vi "Calibration.vi"(8 "error in (no error)":errorcluster) -> (0 "error out":errorcluster, 3 "V 2Pi\nActual":sgl=3.4309938 format="%#.1g")   [LabVIEW 2020]
uses:
  Controls/Calib states --- typedef.ctl
  <vilib>/vision/driver/NI_Vision_Acquisition_Software.lvlib
  <vilib>/vision/NI_Vision_Development_Module.lvlib
  Controls/Calib data ---typedef.ctl
  <vilib>/vision/Image Controls.llb/IMAQ Image.ctl
  64c00cdc-7401-4ced-a99b-d285ba44592a.vi
  Controls/Calibration color ---typedef.ctl
  Controls/LED panel ---typedef.ctl
  <vilib>/userDefined/High Color/IMAQdx.ctl
  Controls/Communication ports ---typedef.ctl
panel:
  out "Voltage range":i32 caption="Max voltage" format="%.0f V"
  out "Current Voltage":dbl format="%0.2f V"
  in  "Piezo voltage":dbl(slide) caption="Initial piezo voltage" min=0.0 max=75.0 step=0.01 scale=0.0..75.0 scale format="%#_2g"
  in  "V range":sgl=0.4 min=0.1 max=75 step=0.1 format="%.1f"
  in  "dt (ms)":i32=50 min=1 max=500 step=1
  in  "LED Panel":T1
  in  "Com ports":T2={"Piezo driver"="MDT694B", "Cam Session"="cam0", "Arduino"="COM7"}
  in  "Sust":bool=TRUE caption="Sustraer?"
  in  "dV (V)":sgl=0.4 min=0.1 max=5 step=0.1 format="%.1f"
  in  "Cancelar":bool
  in  "V 2Pi\nApriori":sgl=4.0 min=0.1 max=15 step=0.1 format="%.1f"
  out "valor enviado":string="17.2"
  in  "Iniciar":bool
  out "Captura":T4(plugin-control)
  out "tiempo total":u32=1016
  out "Ciclos 2Pi":cluster{"xi used":dbl[], "yi":dbl[]}[](graph)=[{"xi used"=[0.0, 0.4000000059604645, 0.800000011920929, 1.2000000476837158, 1.600000023841858, 2.0, 2.4000000953674316, 2.799999952316284, 3.200000047683716, 3.6000001430511475, 4.0, 4.400000095367432, 4.800000190734863, 5.200000286102295, 5.599999904632568, 6.0, 6.400000095367432, 6.800000190734863, 7.200000286102295], "yi"=[1.6194082498550415, 2.081223726272583, 3.9639101028442383, 5.417988300323486, 5.994996547698975, 5.763517379760742, 4.927460193634033, 3.268064022064209, 1.9228070974349976, 2.006049633026123, 3.322584629058838, 5.178757190704346, 5.874281883239746, 5.9817633628845215, 5.3586106300354, 3.7743194103240967, 2.4187028408050537, 2.3153183460235596, 3.7917206287384033]}, {"xi used"=[0.0, 0.10000000149011612, 0.20000000298023224, 0.30000000447034836, 0.4000000059604645, 0.5000000074505806, 0.6000000089406967, 0.7000000104308128, 0.800000011920929, 0.9000000208616257, 1.0000000298023224, 1.100000038743019, 1.2000000476837158, 1.3000000417232513, 1.4000000357627869, 1.5000000298023224, 1.600000023841858, 1.7000000178813934, 1.800000011920929, 1.9000000059604645, 2.0, 2.100000023841858, 2.200000047683716, 2.3000000715255737, 2.4000000953674316, 2.5000000596046448, 2.600000023841858, 2.699999988079071, 2.799999952316284, 2.899999976158142, 3.0, 3.100000023841858, 3.200000047683716, 3.3000000715255737, 3.4000000953674316, 3.5000001192092896, 3.6000001430511475, 3.7000001072883606, 3.8000000715255737, 3.900000035762787, 4.0, 4.100000023841858, 4.200000047683716, 4.300000071525574, 4.400000095367432, 4.5000001192092896, 4.6000001430511475, 4.700000166893005, 4.800000190734863, 4.900000214576721, 5.000000238418579, 5.100000262260437, 5.200000286102295, 5.300000190734863, 5.400000095367432, 5.5, 5.599999904632568, 5.699999928474426, 5.799999952316284, 5.899999976158142, 6.0, 6.100000023841858, 6.200000047683716, 6.300000071525574, 6.400000095367432, 6.5000001192092896, 6.6000001430511475, 6.700000166893005, 6.800000190734863, 6.900000214576721, 7.000000238418579, 7.100000262260437, 7.200000286102295], "yi"=[1.6194082498550415, 1.6415202646400873, 1.700969021152869, 1.835091261121122, 2.081223726272583, 2.4615675244221595, 2.9377812277334487, 3.4563877744572187, 3.9639101028442383, 4.416314498578613, 4.807340439884618, 5.1401707620402455, 5.417988300323486, 5.643229129866736, 5.815342479071086, 5.9330308007455095, 5.994996547698975, 6.0015645873541725, 5.959549445588673, 5.8773880628937665, 5.763517379760742, 5.622745854472534, 5.4453682711596425, 5.218050945615625, 4.927460193634033, 4.566549653810085, 4.153420905030226, 3.7124627576598135, 3.268064022064209, 2.8442846434260165, 2.4638706226251452, 2.1492390703865025, 1.9228070974349976, 1.8016579460584699, 1.7815393847964844, 1.8528653137515367, 2.006049633026123, 2.2327082258196134, 2.529265762805696, 2.8933489839101707, 3.322584629058838, 3.807336769827714, 4.308917005977046, 4.78137419407865, 5.178757190704346, 5.467236063197128, 5.661465721984701, 5.788222288265946, 5.874281883239746, 5.940712665430707, 5.985750942666336, 6.001925060099863, 5.9817633628845215, 5.9173299887642, 5.798831744986865, 5.616011126946077, 5.3586106300354, 5.0225638976458455, 4.628571701943094, 4.203526165358669, 3.7743194103240967, 3.3657338746848104, 2.994113257941885, 2.673691575010305, 2.4187028408050537, 2.2430304554985607, 2.1591553602930404, 2.1792078816481535, 2.3153183460235596, 2.5722541809073114, 2.925331217901028, 3.3425023896347215, 3.7917206287384033]}, {"xi used"=[1.6635191881348852, 5.094512955533968], "yi"=[6.004797437208987, 6.001979760925586]}]
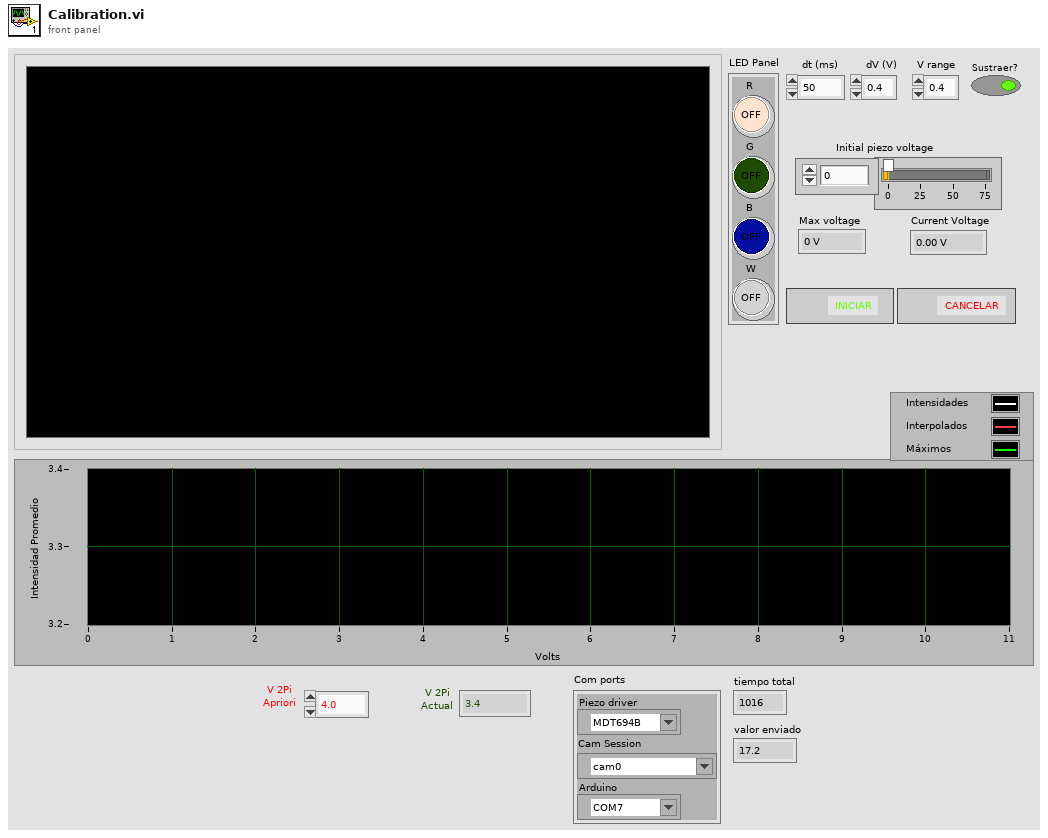
[diagram p1: front panel]
types:
  T1 = typedef "LED panel ---typedef.ctl" = cluster{"R":bool, "G":bool, "B":bool, "W":bool}
  T2 = typedef "Communication ports ---typedef.ctl" = cluster{"Piezo driver":refnum<visa-resource-name>, "Cam Session":T3, "Arduino":refnum<visa-resource-name>}
  T3 = typedef "IMAQdx.ctl" = refnum<k21>
  T4 = typedef "IMAQ Image.ctl" = refnum<image>
  T5 = typedef "Calib data ---typedef.ctl" = cluster{"t0":u32, "Voltage":sgl[], "Mean pix value":sgl[], "Rectangle":cluster{"Left":i32, "Top":i32, "Right":i32, "Bottom":i32}, "New calibration?":bool, "Images":T4[], "Calib color":T6, "Current voltage":sgl}
  T6 = typedef "Calibration color ---typedef.ctl" = enum16{"Red", "Green", "Blue", "White"}
  T7 = typedef "Calib states --- typedef.ctl" = enum16{"Init", "Wait", "Acquire base image", "Aquire and process", "Calculate results", "Clear UI", "Prompt to repeat", "Clear buffers", "Exit"}
  T8 = cluster{"Left":i32, "Top":i32, "Right":i32, "Bottom":i32}
  T9 = typedef "lveventtype.ctl" = enum32{"Null", "Timeout", "Annotation Menu Selection", "Annotation Menu Selection?", "App Instance Close", "App Instance Close?", "Autoscale Range Change", "Bookmark Info Change", "Cell Edit", "Cell Edit?", "Cursor Grab", "Cursor Grab?", "Cursor Menu Selection", "Cursor Menu Selection?", "Cursor Move", "Cursor Release", "Data Change", "Direction Change", "Display State Change", "Drag Ended", "Drag Enter", "Drag Leave", "Drag Over", "Drag Source Update", "Drag Starting", "Drag Starting?", "Drop", "Exec State Change", "Key Down", "Key Down?", "Key Repeat", "Key Repeat?", "Key Up", "Listbox Double Click", "Menu Activation?", "Menu Selection (App)", "Menu Selection? (App)", "Menu Selection (User)", "Mouse Down", "Mouse Down?", "Mouse Enter", "Mouse Leave", "Mouse Move", "Mouse Up", "Mouse Wheel", "NI Security User Change (App)", "Pane Size", "Panel Close", "Panel Close?", "Panel Resize", "Plot Attribute Change", "Scale Range Change", "Shortcut Menu Activation?", "Shortcut Menu Selection (App)", "Shortcut Menu Selection? (App)", "Shortcut Menu Selection (User)", "Tree Double Click", "Tree Drag", "Tree Drag?", "Tree Drop", "Tree Drop?", "Tree Item Close", "Tree Item Close?", "Tree Item Open", "Tree Item Open?", "User Event", "Value Change"}
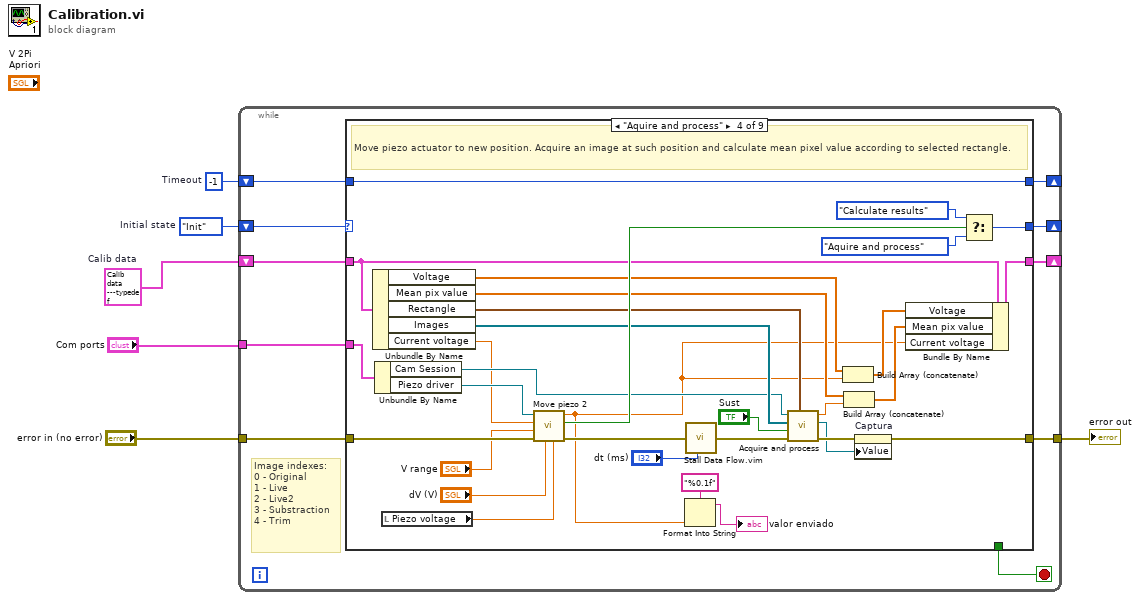
[diagram p0: block diagram]
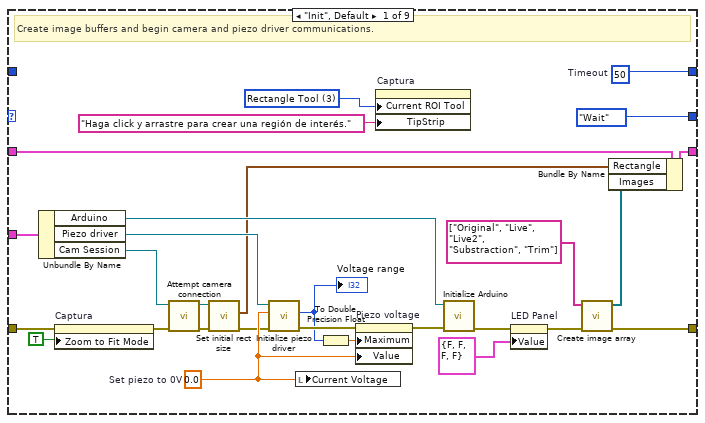
[diagram p2: hidden frame]
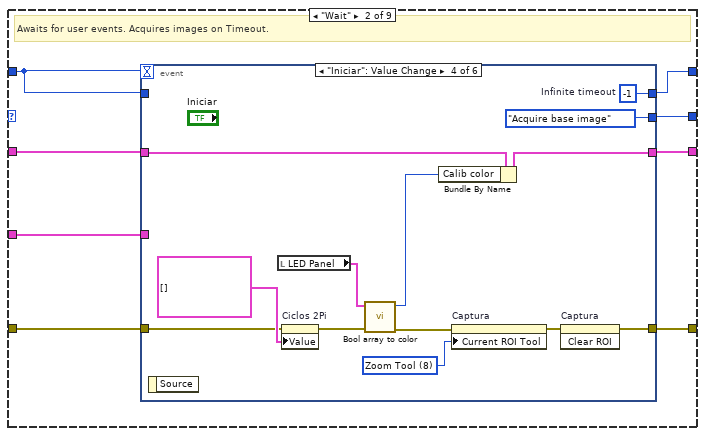
[diagram p3: hidden frame]
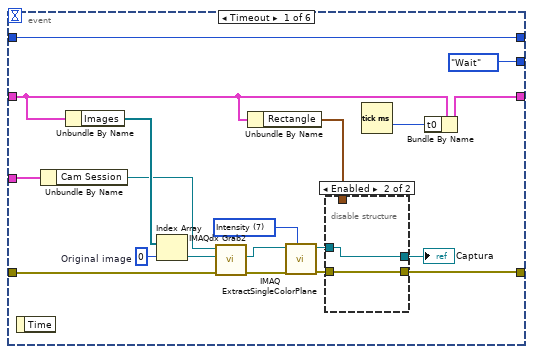
[diagram p4: hidden frame]
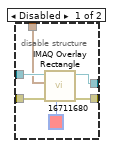
[diagram p5: hidden frame]
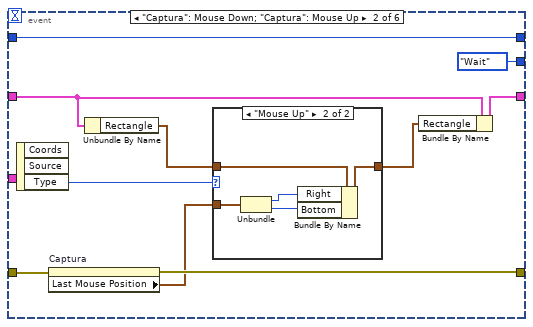
[diagram p6: hidden frame]
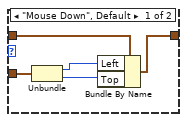
[diagram p7: hidden frame]
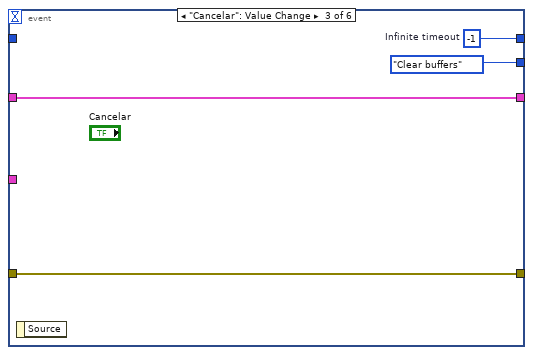
[diagram p8: hidden frame]
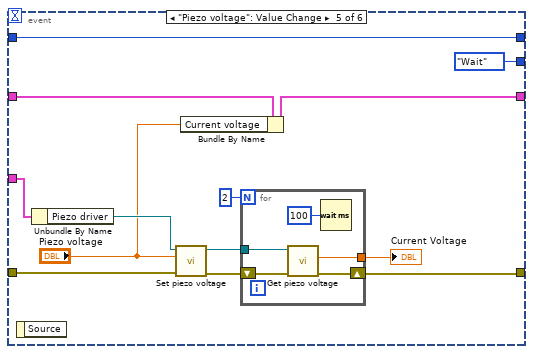
[diagram p9: hidden frame]
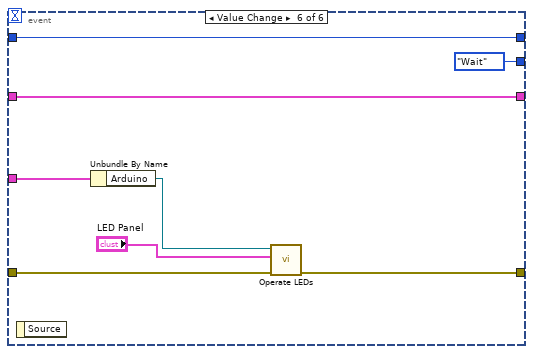
[diagram p10: hidden frame]
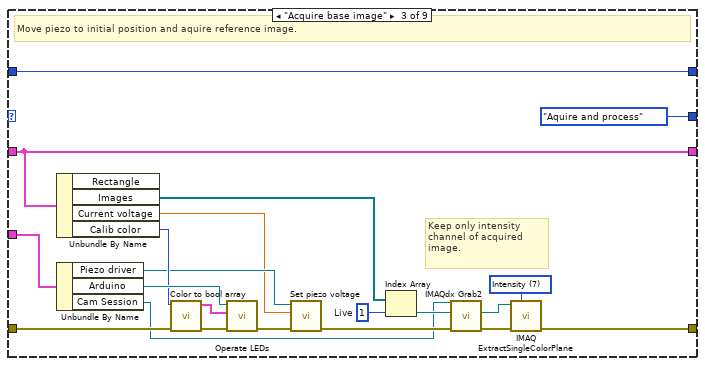
[diagram p11: hidden frame]
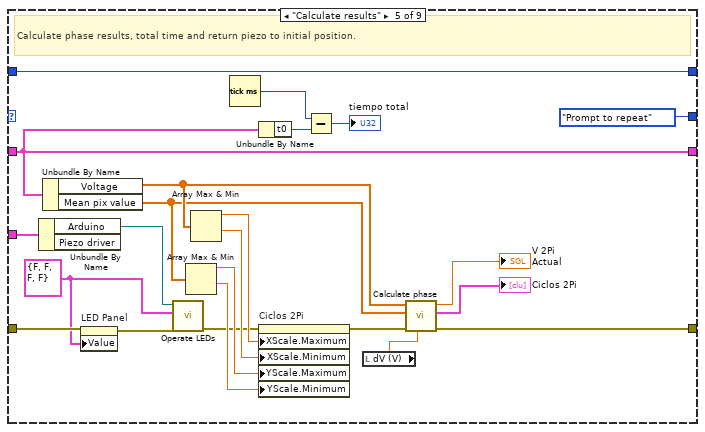
[diagram p12: hidden frame]
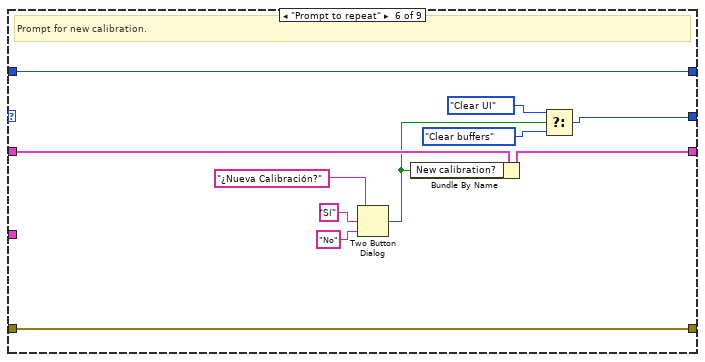
[diagram p13: hidden frame]
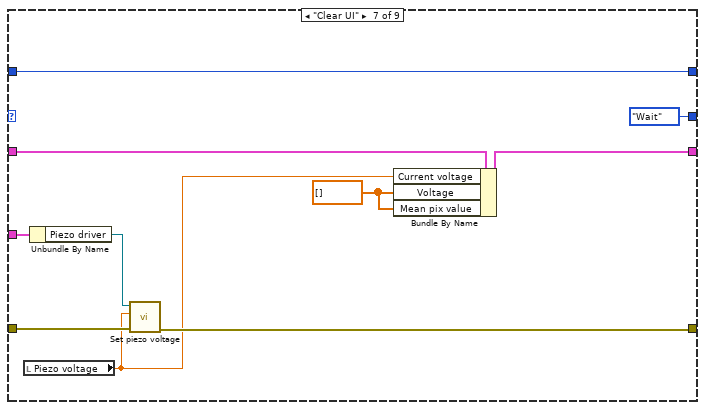
[diagram p14: hidden frame]
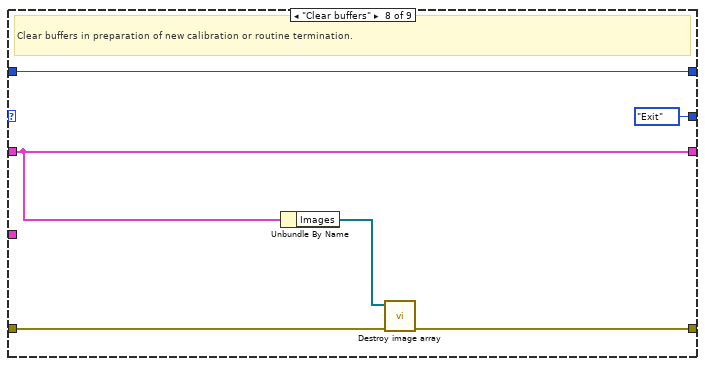
[diagram p15: hidden frame]
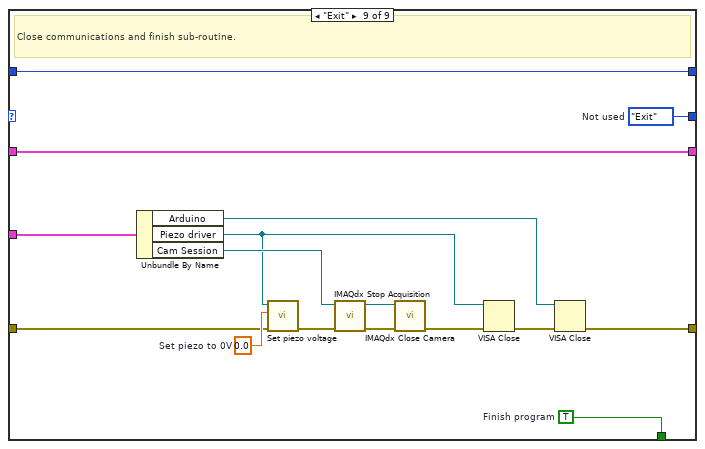
[diagram p16: hidden frame]
diagram:
  w2 = T5 {"t0"=0, "Voltage"=[], "Mean pix value"=[], "Rectangle"={"Left"=0, "Top"=0, "Right"=0, "Bottom"=0}, "New calibration?"=FALSE, "Images"=[], "Calib color"=enum."Red", "Current voltage"=0.0}  # Calib data
  w3 = -1  # Timeout
  w6 = Calib_states_---_typedef."Init"  # Initial state
  n1 = while {
    tunnel: [w14] -> w4
    tunnel: "error in (no error)" -> [w13]
    shift-right: [w12] -> _
    shift-left: w6 -> [w16]
    shift-right: [w10] -> _
    shift-left: w3 -> [w11]
    shift-right: [w9] -> _
    shift-left: w2 -> [w8]
    tunnel: "Com ports" -> [w7]
    stop <- w15 stop-if-true
    # "Image indexes:\n0 - Original\n1 - Live\n2 - Live2\n3 - Substraction\n4 - Trim"
    n2 = case shown="\"Aquire and process\"" w16 {
      tunnel: [_ _ _ _ _ _ _ _ w261] -> w15
      tunnel: [w39 w48 w145 w165 w202 w229 w234 w244 w247] -> w14
      tunnel: w13 -> [w42 w49 w153 w194 w199 w229 w237 w245 w251]
      tunnel: [Calib_states_---_typedef."Wait" w52 Calib_states_---_typedef."Aquire and process" ("Not used") w191 Calib_states_---_typedef."Prompt to repeat" ("Not used") w219 Calib_states_---_typedef."Wait" ("Not used") Calib_states_---_typedef."Exit" ("Not used") w260] -> w12
      tunnel: w11 -> [_ w51 w163 w195 w218 w228 w239 w243 w259]
      tunnel: [w43 w50 w163 w195 w218 w228 w239 w243 w259] -> w10
      tunnel: [w37 w47 w156 w188 w196 w223 w232 w242 w258] -> w9
      tunnel: w8 -> [w38 w46 w156 w187 w196 w224 w233 w242 w258]
      tunnel: w7 -> [w33 w45 w155 w175 w203 _ w236 _ w254]
      frame "Init", Default {
        w21 = 0.0  # Set piezo to 0V
        w35 = u32 3 items=["Zoom Tool"=8, "Selection Tool"=0, "Pan Tool"=9, "Point Tool"=1, "Line Tool"=2, "Rectangle Tool"=3, "Rotated Rectangle Tool"=12, "Polyline Tool"=10, "Polygon Tool"=5, "Freehand Tool"=11, "Closed Freehand Tool"=6, "Ellipse Tool"=4, "Annulus Tool"=7] ("Current ROI Tool")
        w43 = 50  # Timeout
        # "Create image buffers and begin camera and piezo driver communications."
        n3 = Unbundle By Name(w33) -> ("Arduino"=w29:refnum<visa-resource-name>, "Piezo driver"=w32:refnum<visa-resource-name>, "Cam Session"=w31:T3)
        n4 = property on="Captura" class="ImageControl"(error in=w42, "Zoom to Fit Mode"=TRUE) -> (error out=w40:errorcluster)  [unwired: 1 in, 1 out]
        n5 = call "Attempt camera connection.vi"("error in (no error)"=w40, "Camera session"=w31) -> ("error out"=w20:errorcluster, "Cam session Out"=w18:T3)  [unwired: 8 in]
        n6 = call "Set initial rect size.vi"("error in (no error)"=w20, "Cam Session"=w18) -> ("error out"=w19:errorcluster, "Rectangle"=w17:T8)  [unwired: 7 in, 1 out]
        n7 = call "Initialize piezo driver.vi"("error in (no error)"=w19, "Set piezo to 0V"=w21, "COM port in"=w32) -> ("error out"=w28:errorcluster, "Voltage range"=w26:i32)  [unwired: 6 in, 1 out]
        "Voltage range" <- w26
        n8 = local write "Current Voltage"(w21) -> ()
        n9 = To Double Precision Float(number=w26) -> (double precision float=w30:dbl)
        n10 = property on="Piezo voltage" class="Slide (strict)"(error in=w28, "Maximum"=w30, "Value"=w21) -> (error out=w27:errorcluster)  [unwired: 1 in, 1 out]
        n11 = property on="Captura" class="ImageControl"("Current ROI Tool"=w35, "TipStrip"="Haga click y arrastre para crear una región de interés." ("Tip Strip")) -> ()  [unwired: 2 in, 2 out]
        n12 = call "Initialize Arduino.vi"("error in (no error)"=w27, "VISA Refnum in"=w29) -> ("error out"=w25:errorcluster)  [unwired: 9 in]
        n13 = property on="LED Panel" class="Clust (strict)"(error in=w25, "Value"=T1 {"R"=FALSE, "G"=FALSE, "B"=FALSE, "W"=FALSE} ("LED Panel")) -> (error out=w24:errorcluster)  [unwired: 1 in, 1 out]
        n14 = call "Create image array.vi"("error in (no error)"=w24, "Name idx"=string[] ["Original", "Live", "Live2", "Substraction", "Trim"]) -> ("error out"=w39:errorcluster, "Image array"=w36:T4[])  [unwired: 8 in]
        n15 = Bundle By Name(cluster=w38, "Rectangle"=w17, "Images"=w36) -> (w37:T5)
      }
      frame "Wait" {
        # "Awaits for user events. Acquires images on Timeout."
        n16 = event shown="[3] \"Iniciar\": Value Change" {
          selector: _ -> [_ _ _ _ _ _]
          dyn-events: _ -> [_ _ _ _ _ _]
          timeout: w51 -> [_ _ _ _ _ _]
          tunnel: [Calib_states_---_typedef."Wait" Calib_states_---_typedef."Wait" Calib_states_---_typedef."Clear buffers" Calib_states_---_typedef."Acquire base image" Calib_states_---_typedef."Wait" Calib_states_---_typedef."Wait"] -> w52
          tunnel: w51 -> [w70 w89 _ _ w129 w142]
          tunnel: [w70 w89 w100 w115 w129 w142] -> w50
          tunnel: w49 -> [w67 w88 w102 w108 w128 w139]
          tunnel: [w63 w87 w102 w112 w126 w136] -> w48
          tunnel: [w59 w82 w101 w110 w117 w141] -> w47
          tunnel: w46 -> [w56 w83 w101 w111 w119 w141]
          tunnel: w45 -> [w54 _ _ _ w125 w140]
          event Timeout {
            w57 = 7 items=["Red", "Green", "Blue", "Hue", "Saturation", "Luminance", "Value", "Intensity"] ("Color Plane")
            w69 = 0  # Original image
            n17 = event-data() -> ()  [unwired: 1 in, 1 out]
            n18 = Unbundle By Name(w54) -> ("Cam Session"=w53:T3)
            n19 = Unbundle By Name(w56) -> ("Images"=w58:T4[])
            n20 = Index Array(array=w58, index=w69) -> (element=w68:T4)
            n21 = call <vilib>:"IMAQdx Grab2.vi"("error in"=w67, "Image In"=w68, "Session In"=w53) -> ("error out"=w64:errorcluster, "Image Out"=w61:T4)  [unwired: 5 in, 2 out]
            n22 = Unbundle By Name(w56) -> ("Rectangle"=w55:T8)
            n23 = call "IMAQ ExtractSingleColorPlane"("Color Plane"=w57, "error in (no error)"=w64, "Image Src"=w61) -> ("error out"=w66:errorcluster, "Image Dst Out"=w65:T4)  [unwired: 7 in]
            n24 = disable-structure shown="Enabled" {
              disable-tunnel: w66 -> [w77 w78]
              disable-tunnel: w65 -> [w76 w79]
              disable-tunnel: [w75 w78] -> w63
              disable-tunnel: [w74 w79] -> w62
              disable-tunnel: w55 -> [w72 _]
              frame Disabled {
                n25 = call "IMAQ Overlay Rectangle"("Color"=u32 16711680, "error in (no error)"=w77, "Rectangle"=w72, "Image"=w76) -> ("error out"=w75:errorcluster, "Image Out"=w74:T4)  [unwired: 6 in]
              }
              frame Enabled {
              }
            }
            "Captura" <- w62
            n26 = Tick Count (ms)() -> (millisecond timer value=w60:u32)
            n27 = Bundle By Name(cluster=w56, "t0"=w60) -> (w59:T5)
          }
          event "Captura": Mouse Down; "Captura": Mouse Up {
            n28 = event-data() -> ("Type"=w86:T9)  [unwired: 1 in, 2 out]
            n29 = property on="Captura" class="ImageControl"(error in=w88) -> (error out=w87:errorcluster, "Last Mouse Position"=w84:cluster{"X":i32, "Y":i32})  [unwired: 1 in, 1 out]
            n30 = Unbundle By Name(w83) -> ("Rectangle"=w85:T8)
            n31 = case shown="\"Mouse Up\"" w86 {
              tunnel: w85 -> [w91 w98]
              tunnel: w84 -> [w92 w99]
              tunnel: [w90 w95] -> w81
              frame "Mouse Down", Default {
                n32 = Unbundle(w92) -> ("X"=w94:i32, "Y"=w93:i32)
                n33 = Bundle By Name(cluster=w91, "Left"=w94, "Top"=w93) -> (w90:T8)
              }
              frame "Mouse Up" {
                n34 = Unbundle(w99) -> ("X"=w97:i32, "Y"=w96:i32)
                n35 = Bundle By Name(cluster=w98, "Right"=w97, "Bottom"=w96) -> (w95:T8)
              }
            }
            n36 = Bundle By Name(cluster=w83, "Rectangle"=w81) -> (w82:T5)
          }
          event "Cancelar": Value Change {
            w100 = -1  # Infinite timeout
            n37 = event-data() -> ()  [unwired: 1 in, 1 out]
          }
          event "Iniciar": Value Change {
            w114 = u32 8 items=["Zoom Tool"=8, "Selection Tool"=0, "Pan Tool"=9, "Point Tool"=1, "Line Tool"=2, "Rectangle Tool"=3, "Rotated Rectangle Tool"=12, "Polyline Tool"=10, "Polygon Tool"=5, "Freehand Tool"=11, "Closed Freehand Tool"=6, "Ellipse Tool"=4, "Annulus Tool"=7] ("Current ROI Tool")
            w115 = -1  # Infinite timeout
            n38 = event-data() -> ()  [unwired: 1 in, 1 out]
            n39 = local read "LED Panel"() -> (w105:T1)
            n40 = property on="Ciclos 2Pi" class="XYGraph (strict)"(error in=w108, "Value"=cluster{"xi used":dbl[], "yi":dbl[]}[] [] ("Ciclos 2Pi")) -> (error out=w107:errorcluster)  [unwired: 1 in, 1 out]
            n41 = call "Bool array to color.vi"("error in (no error)"=w107, "LED Panel"=w105) -> ("error out"=w106:errorcluster, "Calib color"=w104:T6)  [unwired: 8 in]
            n42 = Bundle By Name(cluster=w111, "Calib color"=w104) -> (w110:T5)
            n43 = property on="Captura" class="ImageControl"(error in=w106, "Current ROI Tool"=w114) -> (error out=w113:errorcluster)  [unwired: 1 in, 1 out]
            n44 = invoke on="Captura" class="ImageControl" method="Clear ROI"(error in=w113) -> (error out=w112:errorcluster)  [unwired: 2 in, 2 out]
          }
          event "Piezo voltage": Value Change {
            n45 = event-data() -> ()  [unwired: 1 in, 1 out]
            n46 = Unbundle By Name(w125) -> ("Piezo driver"=w124:refnum<visa-resource-name>)
            n47 = call "Set piezo voltage.vi"("error in (no error)"=w128, "Voltage"="Piezo voltage", "COM port in"=w124) -> ("error out"=w127:errorcluster, "COM port out"=w123:refnum<visa-resource-name>)  [unwired: 7 in]
            n48 = Bundle By Name(cluster=w119, "Current voltage"="Piezo voltage") -> (w117:T5)
            n49 = for {
              N: 2 -> [_]
              tunnel: w123 -> [w132]
              tunnel: [w131] -> w121
              shift-right: [w133] -> w126
              shift-left: w127 -> [w134]
              n50 = call "Get piezo voltage.vi"("error in (no error)"=w134, "COM port in"=w132) -> ("error out"=w133:errorcluster, "Piezo Voltage"=w131:dbl)  [unwired: 7 in, 1 out]
              n51 = Wait (ms)(milliseconds to wait=u32 100) -> ()  [unwired: 1 out]
            }
            "Current Voltage" <- w121
          }
          event Value Change {
            n52 = event-data() -> ()  [unwired: 1 in, 1 out]
            n53 = Unbundle By Name(w140) -> ("Arduino"=w138:refnum<visa-resource-name>)
            n54 = call "Operate LEDs.vi"("error in (no error)"=w139, "LED Panel"="LED Panel", "COM port in"=w138) -> ("error out"=w136:errorcluster)  [unwired: 7 in, 1 out]
          }
        }
      }
      frame "Acquire base image" {
        w159 = 7 items=["Red", "Green", "Blue", "Hue", "Saturation", "Luminance", "Value", "Intensity"] ("Color Plane")
        w158 = 1  # Live
        # "Keep only intensity channel of acquired image."
        # "Move piezo to initial position and aquire reference image."
        n55 = Unbundle By Name(w156) -> ("Images"=w143:T4[], "Current voltage"=w146:sgl, "Calib color"=w151:T6)  [unwired: 1 out]
        n56 = Unbundle By Name(w155) -> ("Piezo driver"=w147:refnum<visa-resource-name>, "Arduino"=w154:refnum<visa-resource-name>, "Cam Session"=w144:T3)
        n57 = call "Color to bool array.vi"("error in (no error)"=w153, "Calib color"=w151) -> ("error out"=w152:errorcluster, "LED Panel 2"=w150:T1)  [unwired: 8 in]
        n58 = call "Operate LEDs.vi"("error in (no error)"=w152, "LED Panel"=w150, "COM port in"=w154) -> ("error out"=w149:errorcluster)  [unwired: 7 in, 1 out]
        n59 = call "Set piezo voltage.vi"("error in (no error)"=w149, "Voltage"=w146, "COM port in"=w147) -> ("error out"=w148:errorcluster)  [unwired: 7 in, 1 out]
        n60 = Index Array(array=w143, index=w158) -> (element=w161:T4)
        n61 = call <vilib>:"IMAQdx Grab2.vi"("error in"=w148, "Image In"=w161, "Session In"=w144) -> ("error out"=w157:errorcluster, "Image Out"=w160:T4)  [unwired: 5 in, 2 out]
        n62 = call "IMAQ ExtractSingleColorPlane"("Color Plane"=w159, "error in (no error)"=w157, "Image Src"=w160) -> ("error out"=w145:errorcluster)  [unwired: 7 in, 1 out]
      }
      frame "Aquire and process" {
        # "Move piezo actuator to new position. Acquire an image at such position and calculate mean pixel value according to selected rectangle."
        n63 = Unbundle By Name(w187) -> ("Voltage"=w186:sgl[], "Mean pix value"=w183:sgl[], "Rectangle"=w184:T8, "Images"=w178:T4[], "Current voltage"=w169:sgl)
        n64 = Unbundle By Name(w175) -> ("Cam Session"=w173:T3, "Piezo driver"=w174:refnum<visa-resource-name>)
        n65 = local read "Piezo voltage"() -> (w164:dbl)
        n66 = call "Move piezo 2.vi"("Initial voltage"=w164, "dV"="dV (V)", "error in (no error)"=w194, "V Range"="V range", "Current voltage in"=w169, "VISA Refnum in"=w174) -> ("error out"=w168:errorcluster, "Stop?"=w190:bool, "Current voltage out"=w166:sgl)  [unwired: 3 in]
        n67 = Format Into String(format string="%0.1f", w166) -> (resulting string=→"valor enviado":string)  [unwired: 2 in, 1 out]
        n68 = call "Stall Data Flow.vim"("value in"=w168, "milliseconds to wait"="dt (ms)") -> ("value out"=w167:errorcluster)  [unwired: 1 out]
        n69 = call "Acquire and process.vi"("Rectangle"=w184, "error in (no error)"=w167, "Substract images?"="Sust", "Image array"=w178, "Cam session"=w173) -> ("error out"=w180:errorcluster, "Trimmed image"=w179:T4, "Mean Value"=w182:sgl)  [unwired: 4 in]
        n70 = Build Array (concatenate)(w186, w166) -> (w185:sgl[])
        n71 = Build Array (concatenate)(w183, w182) -> (w181:sgl[])
        n72 = property on="Captura" class="ImageControl"(error in=w180, "Value"=w179) -> (error out=w165:errorcluster)  [unwired: 1 in, 1 out]
        n73 = Bundle By Name(cluster=w187, "Voltage"=w185, "Mean pix value"=w181, "Current voltage"=w166) -> (w188:T5)
        n74 = Select(t=Calib_states_---_typedef."Calculate results" ("Not used"), s=w190, f=Calib_states_---_typedef."Aquire and process") -> (s? t:f=w191:T7)
      }
      frame "Calculate results" {
        w197 = T1 {"R"=FALSE, "G"=FALSE, "B"=FALSE, "W"=FALSE} ("LED Panel")
        # "Calculate phase results, total time and return piezo to initial position."
        n75 = Unbundle By Name(w203) -> ("Arduino"=w200:refnum<visa-resource-name>)  [unwired: 1 out]
        n76 = Unbundle By Name(w196) -> ("Voltage"=w209:sgl[], "Mean pix value"=w206:sgl[])
        n77 = property on="LED Panel" class="Clust (strict)"(error in=w199, "Value"=w197) -> (error out=w198:errorcluster)  [unwired: 1 in, 1 out]
        n78 = call "Operate LEDs.vi"("error in (no error)"=w198, "LED Panel"=w197, "COM port in"=w200) -> ("error out"=w201:errorcluster)  [unwired: 7 in, 1 out]
        n79 = Array Max & Min(array=w206) -> (max value=w205:sgl, min value=w204:sgl)  [unwired: 2 out]
        n80 = Array Max & Min(array=w209) -> (max value=w208:sgl, min value=w207:sgl)  [unwired: 2 out]
        n81 = Tick Count (ms)() -> (millisecond timer value=w213:u32)
        n82 = Unbundle By Name(w196) -> ("t0"=w212:u32)
        n83 = property on="Ciclos 2Pi" class="XYGraph (strict)"(error in=w201, "XScale.Maximum"=w208, "XScale.Minimum"=w207, "YScale.Maximum"=w205, "YScale.Minimum"=w204) -> (error out=w210:errorcluster)  [unwired: 1 in, 1 out]
        n84 = Subtract(x=w213, y=w212) -> (x-y=→"tiempo total":u32)
        n85 = local read "dV (V)"() -> (w215:sgl)
        n86 = call "Calculate phase.vi"("dV (V)"=w215, "error in (no error)"=w210, "Mean values"=w206, "Voltages"=w209) -> ("error out"=w202:errorcluster, "Ciclos 2Pi 2"=→"Ciclos 2Pi":cluster{"xi used":dbl[], "yi":dbl[]}[], "V 2Pi\nActual 2"=→"V 2Pi\nActual":sgl)  [unwired: 5 in]
      }
      frame "Prompt to repeat" {
        # "Prompt for new calibration."
        n87 = Two Button Dialog(message="¿Nueva Calibración?", 1:"No" ("F button name (\"Cancel\")"), 2:"Sí" ("F button name (\"Cancel\")")) -> (T button?=w222:bool)
        n88 = Bundle By Name(cluster=w224, "New calibration?"=w222) -> (w223:T5)
        n89 = Select(t=Calib_states_---_typedef."Clear UI", s=w222, f=Calib_states_---_typedef."Clear buffers") -> (s? t:f=w219:T7)
      }
      frame "Clear UI" {
        w230 = sgl[] [] ("Voltage")
        n90 = local read "Piezo voltage"() -> (w231:dbl)
        n91 = Unbundle By Name(w236) -> ("Piezo driver"=w235:refnum<visa-resource-name>)
        n92 = call "Set piezo voltage.vi"("error in (no error)"=w237, "Voltage"=w231, "COM port in"=w235) -> ("error out"=w234:errorcluster)  [unwired: 7 in, 1 out]
        n93 = Bundle By Name(cluster=w233, "Current voltage"=w231, "Voltage"=w230, "Mean pix value"=w230) -> (w232:T5)
      }
      frame "Clear buffers" {
        # "Clear buffers in preparation of new calibration or routine termination."
        n94 = Unbundle By Name(w242) -> ("Images"=w241:T4[])
        n95 = call "Destroy image array.vi"("error in (no error)"=w245, "Image array"=w241) -> ("error out"=w244:errorcluster)  [unwired: 9 in]
      }
      frame "Exit" {
        w252 = 0.0  # Set piezo to 0V
        w260 = Calib_states_---_typedef."Exit"  # Not used
        w261 = TRUE  # Finish program
        # "Close communications and finish sub-routine."
        n96 = Unbundle By Name(w254) -> ("Arduino"=w246:refnum<visa-resource-name>, "Piezo driver"=w249:refnum<visa-resource-name>, "Cam Session"=w253:T3)
        n97 = call "Set piezo voltage.vi"("error in (no error)"=w251, "Voltage"=w252, "COM port in"=w249) -> ("error out"=w250:errorcluster)  [unwired: 7 in, 1 out]
        n98 = call <vilib>:"IMAQdx Stop Acquisition.vi"("error in"=w250, "Session In"=w253) -> ("error out"=w257:errorcluster, "Session Out"=w256:T3)  [unwired: 8 in]
        n99 = call <vilib>:"IMAQdx Close Camera.vi"("error in"=w257, "Session In"=w256) -> ("error out"=w255:errorcluster)  [unwired: 9 in]
        n100 = VISA Close(VISA resource name=w249, error in (no error)=w255) -> (error out=w248:errorcluster)
        n101 = VISA Close(VISA resource name=w246, error in (no error)=w248) -> (error out=w247:errorcluster)
      }
    }
  }
  "error out" <- w4
